vi "ex_BackUpExistFileTDM.vi"(8 "error in":errorcluster, 11 "file path":path) -> (0 "error out":errorcluster, 3 "dup file path":path)   [LabVIEW 2020]
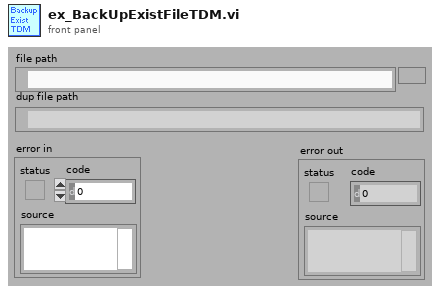
[diagram p1: front panel]
types:
  T1 = enum16{"open", "replace", "create", "open or create", "replace or create", "replace or create with confirmation"}
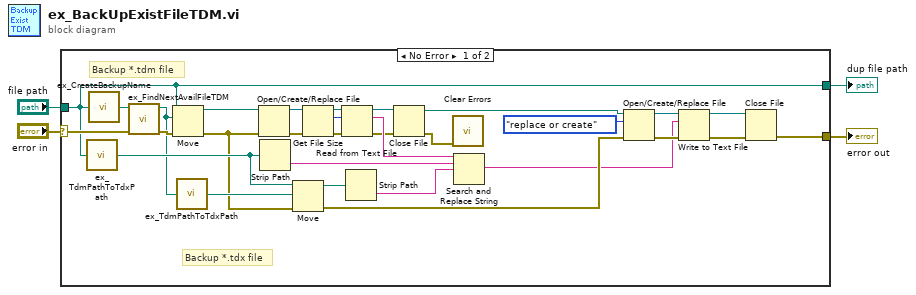
[diagram p0: block diagram]
diagram:
  n1 = case shown="No Error" "error in" {
    selector: "error in" -> [w34 w36]
    tunnel: [w28 w36] -> w3
    tunnel: "file path" -> [w27 w35]
    tunnel: [w27 w35] -> w1
    frame No Error {
      # "Backup *.tdm file"
      # "Backup *.tdx file"
      n2 = call "ex_TdmPathToTdxPath.vi"("TDM path"=w27) -> ("TDX path"=w26:path)
      n3 = call "ex_CreateBackupName.vi"("original name"=w27) -> ("backup name"=w33:path)  [unwired: 4 out]
      n4 = call "ex_FindNextAvailFileTDM.vi"("error in"=w34, "desired file path"=w33) -> ("error out"=w32:errorcluster, "next avail file path"=w25:path)  [unwired: 8 out]
      n5 = Move(source path=w27, error in=w32, 10:w25) -> (error out=w22:errorcluster, 3:w23:path)  [unwired: 3 out]
      n6 = call "ex_TdmPathToTdxPath.vi"("TDM path"=w25) -> ("TDX path"=w24:path)
      n7 = Open/Create/Replace File(file path (use dialog)=w23, error in=w22) -> (refnum out=w9:refnum<file>, error out=w8:errorcluster)  [unwired: 5 out]
      n8 = Strip Path(path=w26) -> (name=w29:string)  [unwired: 1 out]
      n9 = Move(source path=w26, error in=w22, 10:w24) -> (error out=w18:errorcluster, 3:w31:path)  [unwired: 3 out]
      n10 = Get File Size(file=w9, error in=w8) -> (refnum out=w6:refnum<file>, size (in bytes)=w5:i64, 0:w7:errorcluster)
      n11 = Read from Text File(file (use dialog)=w6, count=w5, error in=w7) -> (refnum out=w20:refnum<file>, text=w21:string, error out=w19:errorcluster)  [unwired: 2 out]
      n12 = Strip Path(path=w31) -> (name=w30:string)  [unwired: 1 out]
      n13 = Close File(refnum=w20, error in=w19) -> (path=w16:path, error out=w10:errorcluster)
      n14 = call "Clear Errors.vi"("error in (no error)"=w10) -> ()  [unwired: 1 in, 6 out]
      n15 = Search and Replace String(input string=w21, search string=w29, replace string=w30) -> (result string=w11:string)  [unwired: 1 in, 7 out]
      n16 = Open/Create/Replace File(file path (use dialog)=w16, error in=w18, operation (0:open)=T1."replace or create") -> (refnum out=w14:refnum<file>, error out=w15:errorcluster)  [unwired: 4 out]
      n17 = Write to Text File(file (use dialog)=w14, text=w11, error in=w15) -> (refnum out=w13:refnum<file>, error out=w12:errorcluster)  [unwired: 2 out]
      n18 = Close File(refnum=w13, error in=w12) -> (error out=w28:errorcluster)  [unwired: 1 out]
    }
    frame Error {
    }
  }
  "error out" <- w3
  "dup file path" <- w1
